vi "mkSetROIs.vi"(10 "Camera in":T1={"Gain [1-4]"=0.0, "Offset"=0, "Mode"=6, "ROIs"=[], "ROI Size"={"X"=0, "Y"=0}, "Number of buffers"=40, "Use hardware multiple-ROI?"=TRUE, "GenericCameraConfig"={"Framerate (Hz)"=60, "Exposure time (us)"=5000, "Image size"={"Width"=1280, "Height"=1024}, "Number of buffers"=30}}, 11 "IMAQ Refnum in":refnum<k11>) -> (3 "IMAQ Refnum out":refnum<k11>)   [LabVIEW 2011]
uses:
  CameraConfig.ctl
  Main/Camera/GenericCameraConfigType.ctl
panel:
  out ":d response":string
  # "us"
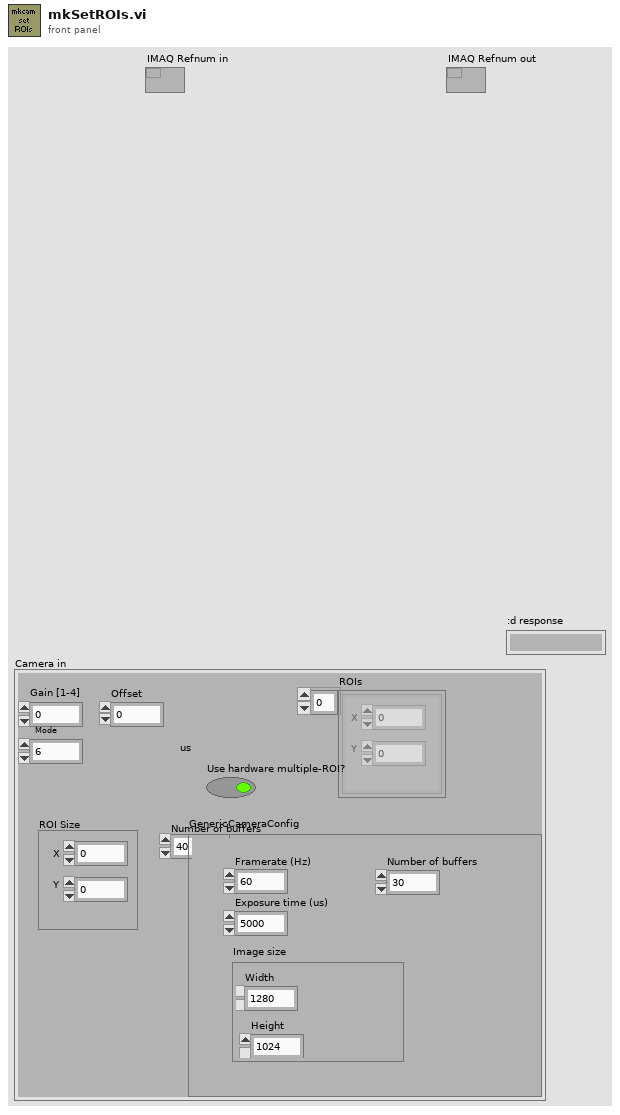
[diagram p1: front panel]
types:
  T1 = typedef "CameraConfig.ctl" = cluster{"Gain [1-4]":sgl, "Offset":i16, "Mode":i16, "ROIs":cluster{"X":i32, "Y":i32}[], "ROI Size":cluster{"X":i32, "Y":i32}, "Number of buffers":i32, "Use hardware multiple-ROI?":bool, "GenericCameraConfig":T2}
  T2 = typedef "GenericCameraConfigType.ctl" = cluster{"Framerate (Hz)":i32, "Exposure time (us)":i32, "Image size":cluster{"Width":i32, "Height":i32}, "Number of buffers":i32}
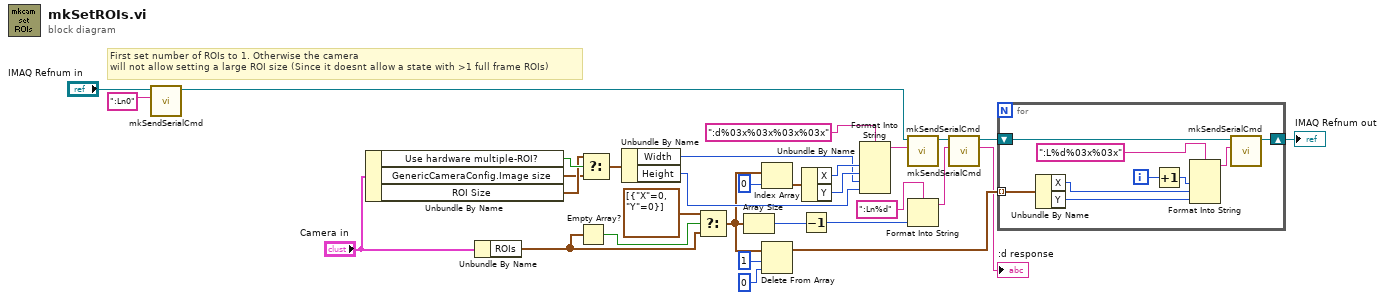
[diagram p0: block diagram]
diagram:
  # "First set number of ROIs to 1. Otherwise the camera\nwill not allow setting a large ROI size (Since it doesnt allow a state with >1 full frame ROIs)"
  n1 = call "mkSendSerialCmd.vi"("String"=":Ln0", "IMAQ Refnum in"="IMAQ Refnum in") -> ("IMAQ Refnum out"=w2:refnum<k11>)  [unwired: 6 in, 3 out]
  n2 = Unbundle By Name("Camera in") -> ("Use hardware multiple-ROI?"=w14:bool, "GenericCameraConfig.Image size"=w11:cluster{"Width":i32, "Height":i32}, "ROI Size"=w12:cluster{"X":i32, "Y":i32})
  n3 = Unbundle By Name("Camera in") -> ("ROIs"=w5:cluster{"X":i32, "Y":i32}[])
  n4 = Empty Array?(array=w5) -> (empty?=w7:bool)
  n5 = Select(t=w12, s=w14, f=w11) -> (s? t:f=w10:cluster{"Width":i32, "Height":i32})
  n6 = Unbundle By Name(w10) -> ("Width"=w9:i32, "Height"=w8:i32)
  n7 = Select(t=cluster{"X":i32, "Y":i32}[] [{"X"=0, "Y"=0}] ("ROIs"), s=w7, f=w5) -> (s? t:f=w4:cluster{"X":i32, "Y":i32}[])
  n8 = Array Size(array=w4) -> (size(s)=w29:i32)
  n9 = Index Array(array=w4, index=0) -> (element=w26:cluster{"X":i32, "Y":i32})
  n10 = Delete From Array(array=w4, length=1 ("index"), index=0) -> (array with subset deleted=w21:cluster{"X":i32, "Y":i32}[])  [unwired: 1 out]
  n11 = Decrement(x=w29) -> (x-1=w31:i32)
  n12 = Unbundle By Name(w26) -> ("X"=w25:i32, "Y"=w24:i32)
  n13 = Format Into String(format string=":d%03x%03x%03x%03x", w25, w24, w9, w8) -> (resulting string=w15:string)  [unwired: 2 in, 1 out]
  n14 = call "mkSendSerialCmd.vi"("String"=w15, "IMAQ Refnum in"=w2) -> ("IMAQ Refnum out"=w19:refnum<k11>)  [unwired: 6 in, 3 out]
  n15 = Format Into String(format string=":Ln%d", w31) -> (resulting string=w16:string)  [unwired: 2 in, 1 out]
  n16 = call "mkSendSerialCmd.vi"("String"=w16, "IMAQ Refnum in"=w19) -> ("String Read"=→":d response":string, "IMAQ Refnum out"=w20:refnum<k11>)  [unwired: 6 in, 2 out]
  n17 = for {
    tunnel: w21 -> [w40] mode=indexing
    shift-right: [w33] -> w17
    shift-left: w20 -> [w34]
    i -> [w38]
    n18 = Unbundle By Name(w40) -> ("X"=w36:i32, "Y"=w35:i32)
    n19 = Increment(x=w38) -> (x+1=w37:i32)
    n20 = Format Into String(format string=":L%d%03x%03x", w37, w36, w35) -> (resulting string=w32:string)  [unwired: 2 in, 1 out]
    n21 = call "mkSendSerialCmd.vi"("String"=w32, "IMAQ Refnum in"=w34) -> ("IMAQ Refnum out"=w33:refnum<k11>)  [unwired: 6 in, 3 out]
  }
  "IMAQ Refnum out" <- w17
